vi "Move Slit Relative.vi"(6 "Target":dbl[unit], 7 "Mono System # (0)":T2, 8 "error in (no error)":errorcluster, 9 "Steps to Move":i32, 10 "Slit (Front/Axial Entrance)":T1, 11 "VISA resource name":refnum<visa-resource-name>) -> (0 "error out":errorcluster, 3 "VISA resource name out":refnum<visa-resource-name>)   [LabVIEW 2023, in "JY-SPEX-TRIAX.lvlib"]
doc: "Moves the spectrometer's slits a relative number of steps from their current position. Returns control immediately (before the slits are done moving).\n\nA positive number of steps opens the slits wider, while a negative makes them narrower. This command corrects for backlash automatically.\n\nOnly one stepper motor can move at a time; thus, this command waits if either other slits or the wavelength drive are being moved.\n\nThe limit to the number of steps that can be moved is the total number of possible steps for the slit."
uses:
  JY-SPEX-TRIAX.lvlib
  controls.llb/Monochromator System Number.ctl
  controls.llb/Slits.ctl
  Spectrometer Config.vi
panel:
  out "Backlash":i32
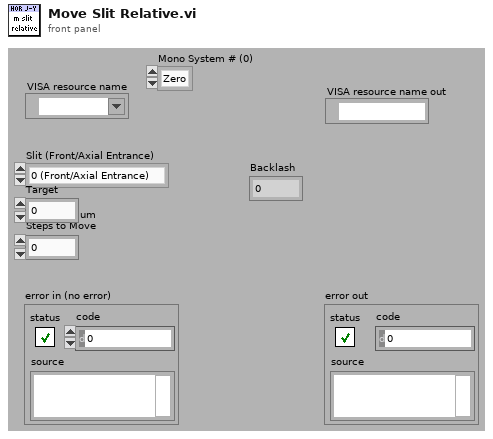
[diagram p1: front panel]
types:
  T1 = typedef "JY-SPEX-TRIAX.lvlib/Slits.ctl" = enum16{"0 (Front/Axial Entrance)", "1 (Side/Lateral Entrance)", "2 (Front/Axial Exit)", "3 (Side/Lateral Exit)"}
  T2 = typedef "JY-SPEX-TRIAX.lvlib/Monochromator System Number.ctl" = enum16{"Zero", "One"}
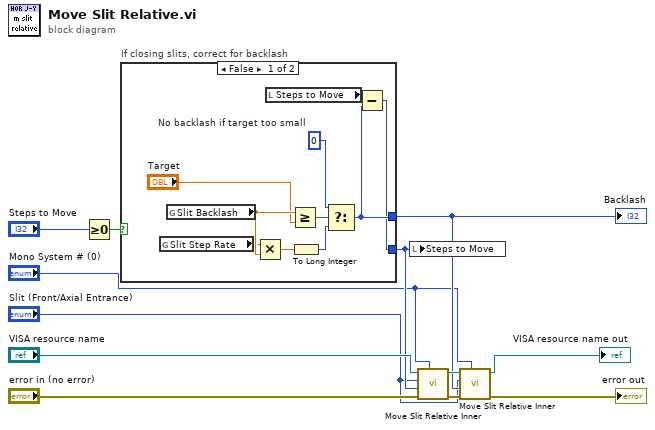
[diagram p0: block diagram]
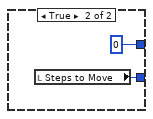
[diagram p2: hidden frame]
diagram:
  n1 = Greater Or Equal To 0?(x="Steps to Move") -> (x >= 0?=w7:bool)
  n2 = case "If closing slits, correct for backlash" shown="False" w7 {
    tunnel: [w19 0 ("f")] -> w3
    tunnel: [w18 w23] -> w4
    frame False {
      w15 = 0  # No backlash if target too small
      n3 = global read "Spectrometer Config.vi" "Slit Step Rate"() -> (w17:dbl[unit])
      n4 = global read "Spectrometer Config.vi" "Slit Backlash"() -> (w22:dbl[unit])
      n5 = Multiply(x=w17, y=w22) -> (x*y=w20:dbl)
      n6 = local read "Steps to Move"() -> (w16:i32)
      n7 = Greater Or Equal?(x=w22, y="Target") -> (x >= y?=w21:bool)
      n8 = To Long Integer(number=w20) -> (32bit integer=w14:i32)
      n9 = Select(t=w15, s=w21, f=w14) -> (s? t:f=w19:i32)
      n10 = Subtract(x=w16, y=w19) -> (x-y=w18:i32)
    }
    frame True {
      n11 = local read "Steps to Move"() -> (w23:i32)
    }
  }
  "Backlash" <- w3
  n12 = local write "Steps to Move"(w4) -> ()
  n13 = call "Move Slit Relative Inner.vi"("Mono System # (0)"="Mono System # (0)", "error in (no error)"="error in (no error)", "Steps to Move"=w4, "Slit (Front/Axial Entrance)"="Slit (Front/Axial Entrance)", "VISA resource name"="VISA resource name") -> ("error out"=w5:errorcluster, "VISA resource name out"=w6:refnum<visa-resource-name>)  [unwired: 5 out]
  n14 = call "Move Slit Relative Inner.vi"("Mono System # (0)"="Mono System # (0)", "error in (no error)"=w5, "Steps to Move"=w3, "Slit (Front/Axial Entrance)"="Slit (Front/Axial Entrance)", "VISA resource name"=w6) -> ("error out"=→"error out":errorcluster, "VISA resource name out"=→"VISA resource name out":refnum<visa-resource-name>)  [unwired: 5 out]
